vi "Update State.vi"(8 "error in (no error)":errorcluster, 10 "samples generated":i32, 11 "signal configuration":refnum<class "SV Discrete Sweep.lvclass">) -> (0 "error out":errorcluster, 1 "segment done":bool, 2 "generation done":bool, 3 "signal configuration":refnum<class "SV Discrete Sweep.lvclass">, 4 "measurement done":bool)   [LabVIEW 2017, in "SV Discrete Sweep.lvclass"]
uses:
  <vilib>/addons/_NISVFA/_Generation/Signal Generation/SV Discrete Sweep/SV Discrete Sweep.lvclass
  C:/Program Files (x86)/National Instruments/LabVIEW 2017/vi.lib/addons/_NISVFA/_Generation/Signal Generation/SV Signal/SV Signal.lvclass
  C:/Program Files (x86)/National Instruments/LabVIEW 2017/vi.lib/addons/_NISVFA/_Generation/Signal Generation/SV Function/SV Function.lvclass
  <vilib>/addons/_NISVFA/_Generation/Signal Generation/SV Signal/sv_Signal State Attribute.ctl
  <vilib>/addons/_NISVFA/_Generation/Signal Generation/SV Signal/sv_Generation State.ctl
  <vilib>/addons/_NISVFA/_Generation/Signal Generation/SV Discrete Sweep/SV Discrete Sweep.lvclass/SV Discrete Sweep.ctl
  <vilib>/addons/_NISVFA/_Generation/subVIs/sv_Optimum Location.ctl
  <vilib>/addons/_NISVFA/_Generation/Signal Generation/SV Signal/SV Signal.lvclass
  <vilib>/addons/_NISVFA/_Generation/Signal Generation/SV Signal/Read Transition Profile.vi
  <vilib>/addons/_NISVFA/_Generation/Signal Generation/SV Function/SV Function.lvclass
  <vilib>/addons/_NISVFA/_Generation/SoundVib_Generation.lvlib
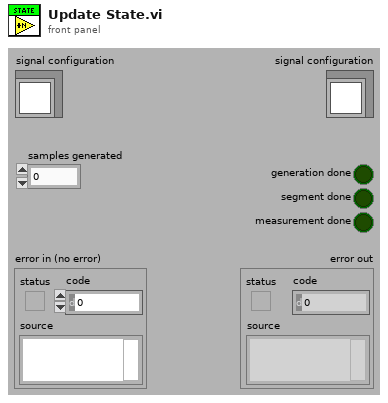
[diagram p1: front panel]
types:
  T1 = typedef "SV Signal.lvclass/sv_Signal State Attribute.ctl" = string
  T2 = typedef "SV Signal.lvclass/sv_Generation State.ctl" = enum16{"Idle", "Ramp Up", "Pre-Measurement Settling", "Measurement", "Post-Measurement Settling", "Discrete Sweep Transition", "Ramp Down", "Update"}
  T3 = typedef "SoundVib_Generation.lvlib/sv_Optimum Location.ctl" = enum16{"Zero Crossing, First Available", "Zero Crossing, Positive Slope", "Zero Crossing, Negative Slope", "Peak or Valley", "Peak", "Valley"}
  T4 = typedef "SV Signal.lvclass/sv_System Timing Model.ctl" = i64
  T5 = cluster{"system timing model":T4, "state":cluster{"RESET":bool, "generator timestamp":timestamp, "elapsed seconds":dbl, "elapsed samples":u64, "generation state":T2, "time offset at state":dbl, "samples generated at state":u64, "signal state":variant}, "duration of state":dbl, "samples remaining at state":i32}
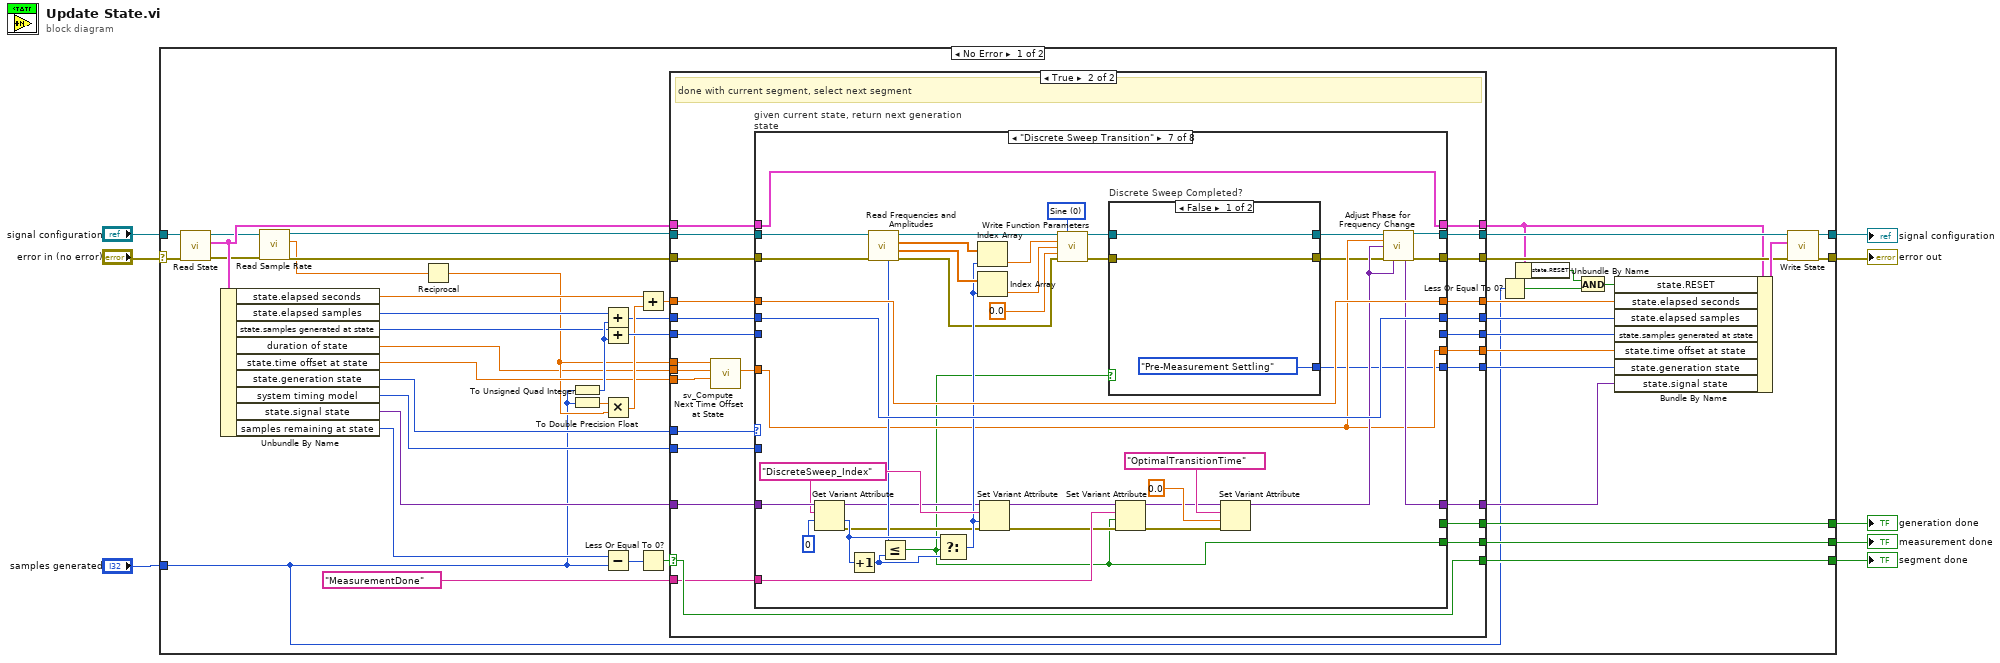
[diagram p0: block diagram]
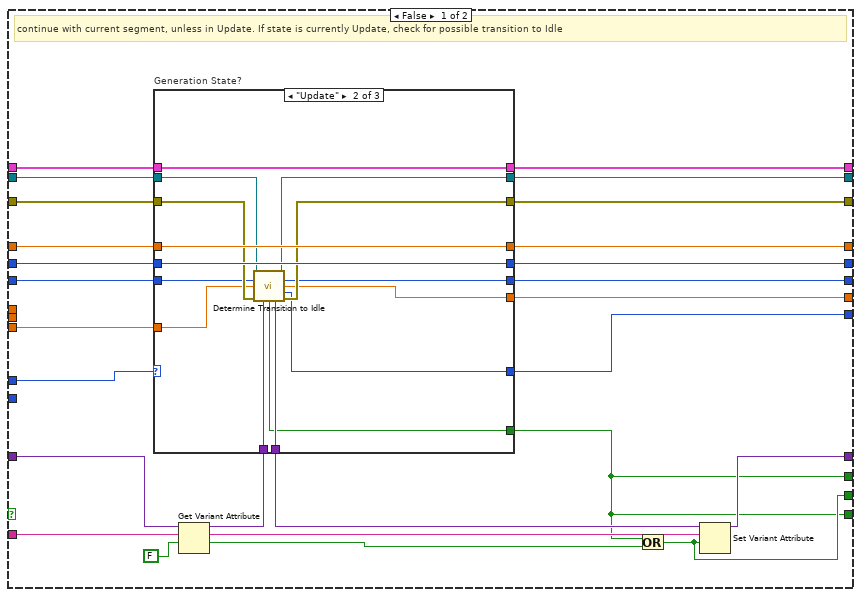
[diagram p2: hidden frame]
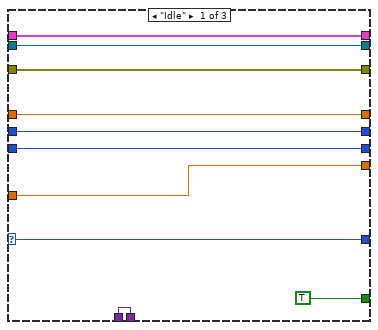
[diagram p3: hidden frame]
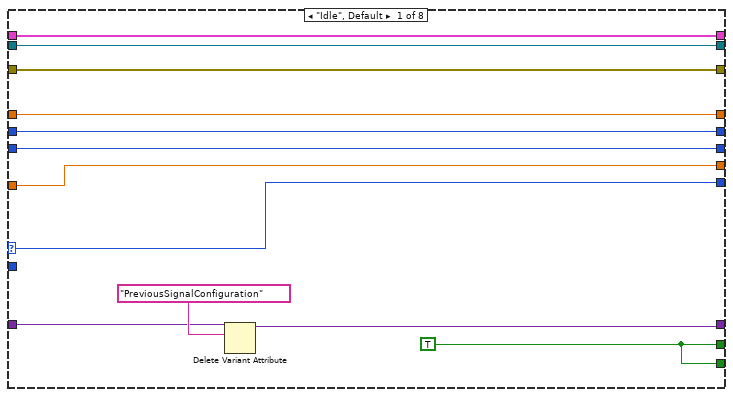
[diagram p5: hidden frame]
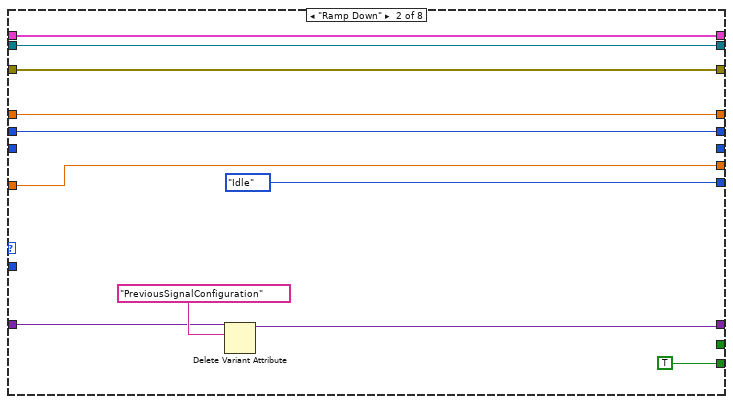
[diagram p6: hidden frame]
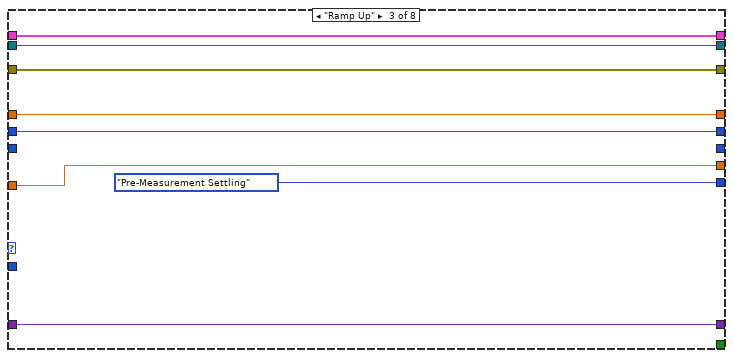
[diagram p7: hidden frame]
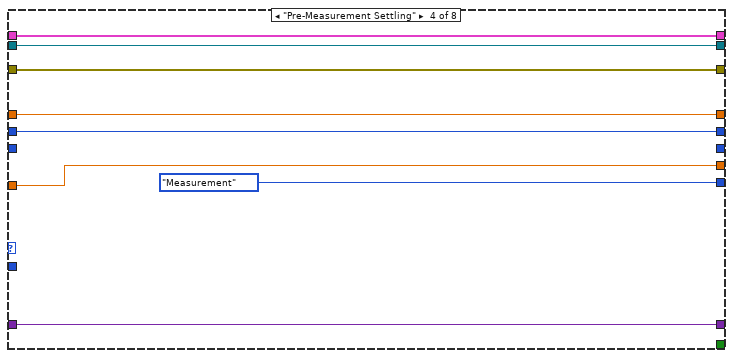
[diagram p8: hidden frame]
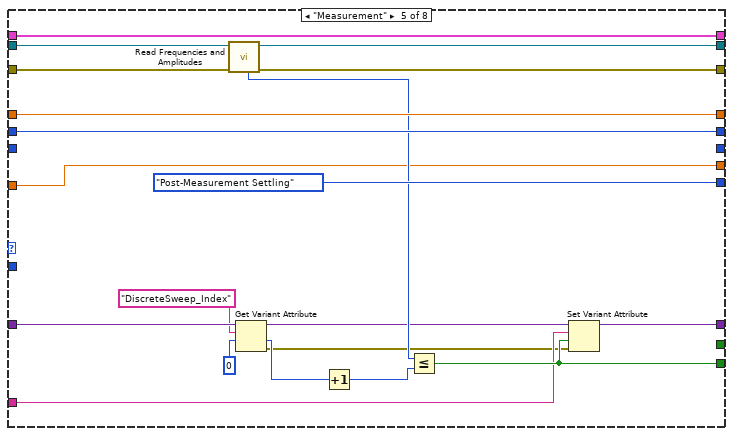
[diagram p9: hidden frame]
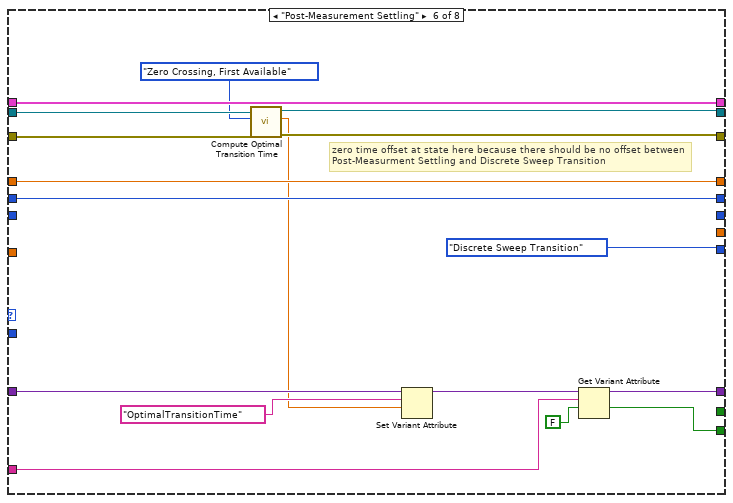
[diagram p10: hidden frame]
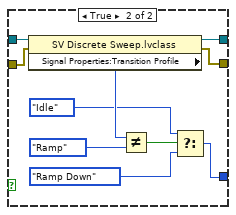
[diagram p11: hidden frame]
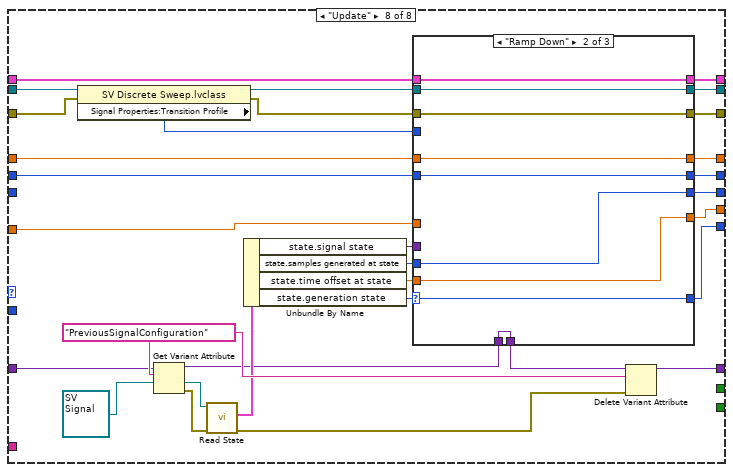
[diagram p12: hidden frame]
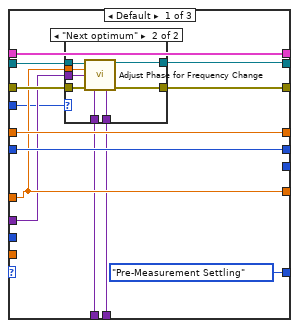
[diagram p13: hidden frame]
diagram:
  n1 = case shown="No Error" "error in (no error)" {
    selector: "error in (no error)" -> [w42 w341]
    tunnel: [w41 w341] -> w4
    tunnel: [w43 w342] -> w8
    tunnel: "signal configuration" -> [w45 w342]
    tunnel: "samples generated" -> [w9 _]
    tunnel: [w25 _] -> w3
    tunnel: [w46 _] -> w1
    tunnel: [w24 _] -> w2
    frame No Error {
      n2 = call <vilib>:"Read State.vi"("error in (no error)"=w42, "signal configuration"=w45) -> ("error out"=w19:errorcluster, "generator state"=w33:T5, "signal configuration"=w22:refnum<class "SV Discrete Sweep.lvclass">)  [unwired: 7 in]
      n3 = Unbundle By Name(w33) -> ("state.elapsed seconds"=w49:dbl, "state.elapsed samples"=w54:u64, "state.samples generated at state"=w39:u64, "duration of state"=w15:dbl, "state.time offset at state"=w17:dbl, "state.generation state"=w48:T2, "system timing model"=w47:T4, "state.signal state"=w36:variant, "samples remaining at state"=w26:i32)
      n4 = call <vilib>:"Read Sample Rate.vi"("error in (no error)"=w19, "signal configuration"=w22) -> ("error out"=w20:errorcluster, "sample rate [Hz]"=w18:dbl, "signal configuration"=w21:refnum<class "SV Discrete Sweep.lvclass">)  [unwired: 7 in]
      n5 = Reciprocal(x=w18) -> (1/x=w16:dbl)
      n6 = To Unsigned Quad Integer(1:w9) -> (0:w40:u64)
      n7 = To Double Precision Float(number=w9) -> (double precision float=w53:dbl)
      n8 = Add(x=w54, y=w40) -> (x+y=w31:u64)
      n9 = Add(x=w39, y=w40) -> (x+y=w38:u64)
      n10 = Multiply(x=w53, y=w16) -> (x*y=w37:dbl)
      n11 = Subtract(x=w26, y=w9) -> (x-y=w51:i32)
      n12 = Add(x=w49, y=w37) -> (x+y=w29:dbl)
      n13 = Less Or Equal To 0?(x=w51) -> (x <= 0?=w52:bool)
      n14 = case "done with segment?" shown="True" w52 {
        selector: w52 -> [_ w135]
        tunnel: [w56 w139] -> w35
        tunnel: w47 -> [_ w138]
        tunnel: w48 -> [w55 w137]
        tunnel: [w57 w136] -> w25
        tunnel: [w62 w120] -> w13
        tunnel: [w63 w119] -> w50
        tunnel: [w57 w135] -> w46
        tunnel: w38 -> [w65 w114]
        tunnel: w17 -> [w64 w115]
        tunnel: w36 -> [w79 w134]
        tunnel: [w78 w133] -> w34
        tunnel: w21 -> [w72 w132]
        tunnel: w33 -> [w73 w122]
        tunnel: w20 -> [w71 w130]
        tunnel: [w61 w126] -> w32
        tunnel: w31 -> [w66 w125]
        tunnel: [w60 w128] -> w30
        tunnel: w29 -> [w67 w127]
        tunnel: [w69 w131] -> w28
        tunnel: [w68 w121] -> w14
        tunnel: [w70 w129] -> w27
        tunnel: [w74 w124] -> w24
        tunnel: T1 "MeasurementDone" ("name") -> [w77 w123]
        tunnel: w16 -> [_ w117]
        tunnel: w15 -> [_ w116]
        frame False {
          # "continue with current segment, unless in Update. If state is currently Update, check for possible transition to Idle"
          n15 = Get Variant Attribute(Variant=w79, name=w77, default value (empty Variant)=FALSE) -> (duplicate Variant=w59:variant, value=w75:bool)  [unwired: 1 in, 2 out]
          n16 = case "Generation State?" shown="\"Update\"" w55 {
            selector: w55 -> [w80 _ w105]
            tunnel: [w89 w95 w113] -> w62
            tunnel: w65 -> [w89 w97 w113]
            tunnel: [w88 w94 w112] -> w63
            tunnel: w64 -> [w88 w96 w112]
            tunnel: [TRUE w90 _] -> w57
            tunnel: [w86 w100 w111] -> w69
            tunnel: w72 -> [w86 w101 w111]
            tunnel: [w85 w104 w110] -> w68
            tunnel: w73 -> [w85 w104 w110]
            tunnel: [w84 w98 w109] -> w70
            tunnel: w71 -> [w84 w99 w109]
            tunnel: [w83 w103 w108] -> w60
            tunnel: w67 -> [w83 w103 w108]
            tunnel: [w82 w102 w107] -> w61
            tunnel: w66 -> [w82 w102 w107]
            tunnel: w59 -> [w81 w93 w106]
            tunnel: [w81 w92 w106] -> w58
            tunnel: [w80 w91 w105] -> w56
            frame "Idle" {
            }
            frame "Update" {
              n17 = call <vilib>:"Determine Transition to Idle.vi"("SV Signal in"=w101, "samples generated at state in"=w97, "time offset at state in"=w96, "error in (no error)"=w99, "signal state in"=w93) -> ("SV Signal out"=w100:refnum<class "SV Discrete Sweep.lvclass">, "samples generated at state out"=w95:u64, "time offset at state out"=w94:dbl, "generation state out"=w91:T2, "transitioned to Idle?"=w90:bool, "signal state out"=w92:variant, "error out"=w98:errorcluster)  [unwired: 4 in]
            }
            frame Default {
            }
          }
          n18 = Or(x=w57, y=w75) -> (x .or. y?=w74:bool)
          n19 = Set Variant Attribute(Variant=w58, name=w77, value=w74) -> (Variant out=w78:variant)  [unwired: 1 in, 2 out]
        }
        frame True {
          # "done with current segment, select next segment"
          n20 = call <vilib>:"sv_Compute Next Time Offset at State.vi"("time offset at previous state"=w115, "duration of previous state"=w116, "dt"=w117) -> ("time offset at next state"=w118:dbl)  [unwired: 8 in]
          n21 = case "given current state, return next generation state" shown="\"Discrete Sweep Transition\"" w137 {
            selector: w137 -> [w141 _ _ _ _ _ _ _]
            tunnel: w138 -> [_ _ _ _ _ _ _ _]
            tunnel: [w141 sv_Generation_State."Idle" ("generation state") sv_Generation_State."Pre-Measurement Settling" ("generation state") sv_Generation_State."Measurement" ("generation state") sv_Generation_State."Post-Measurement Settling" ("generation state") sv_Generation_State."Discrete Sweep Transition" ("generation state") w216 w291] -> w139
            tunnel: [w147 _ _ _ _ _ _ _] -> w136
            tunnel: w134 -> [w145 w155 w169 w177 w197 w202 w255 w296]
            tunnel: [w144 w154 w169 w177 w194 w212 w225 w299] -> w133
            tunnel: w132 -> [w151 w161 w168 w176 w187 w208 w223 w273]
            tunnel: [w151 w161 w168 w176 w186 w207 w228 w284] -> w131
            tunnel: w130 -> [w150 w160 w167 w175 w185 w206 w222 w272]
            tunnel: [w150 w160 w167 w175 w184 w205 w227 w283] -> w129
            tunnel: [w149 w159 w166 w174 w196 w214 w253 w281] -> w128
            tunnel: w127 -> [w149 w159 w166 w174 w196 w214 w253 w282]
            tunnel: [w148 w158 w165 w173 w195 w213 w252 w280] -> w126
            tunnel: w125 -> [w148 w158 w165 w173 w195 w213 w252 w279]
            tunnel: [w147 TRUE _ _ w193 w209 w221 _] -> w124
            tunnel: w123 -> [_ _ _ _ w192 w211 w251 _]
            tunnel: w122 -> [w143 w153 w164 w172 w180 w204 w233 w285]
            tunnel: [w143 w153 w164 w172 w180 w204 w233 w286] -> w121
            tunnel: [w140 _ _ _ _ _ _ w292] -> w120
            tunnel: [w142 w152 w163 w171 w179 _ w224 w288] -> w119
            tunnel: w118 -> [w142 w152 w163 w171 w179 _ w224 w287]
            tunnel: w114 -> [w140 _ _ _ _ _ _ _]
            frame "Idle", Default {
              w147 = TRUE
              n22 = Delete Variant Attribute(6:T1 "PreviousSignalConfiguration" ("name (all attributes)"), 7:w145) -> (3:w144:variant)  [unwired: 1 in, 2 out]
            }
            frame "Ramp Down" {
              n23 = Delete Variant Attribute(6:T1 "PreviousSignalConfiguration" ("name (all attributes)"), 7:w155) -> (3:w154:variant)  [unwired: 1 in, 2 out]
            }
            frame "Ramp Up" {
            }
            frame "Pre-Measurement Settling" {
            }
            frame "Measurement" {
              n24 = call <vilib>:"Read Frequencies and Amplitudes.vi"("error in (no error)"=w185, "SV Discrete Sweep in"=w187) -> ("error out"=w184:errorcluster, "SV Discrete Sweep out"=w186:refnum<class "SV Discrete Sweep.lvclass">, "number of steps"=w183:i32)  [unwired: 5 in, 2 out]
              n25 = Get Variant Attribute(Variant=w197, name="DiscreteSweep_Index", default value (empty Variant)=0 ("samples generated")) -> (duplicate Variant=w182:variant, value=w190:i32, error out=w181:errorcluster)  [unwired: 1 in, 1 out]
              n26 = Increment(x=w190) -> (x+1=w189:i32)
              n27 = Less Or Equal?(x=w183, y=w189) -> (x <= y?=w193:bool)
              n28 = Set Variant Attribute(Variant=w182, name=w192, value=w193, error in=w181) -> (Variant out=w194:variant)  [unwired: 2 out]
            }
            frame "Post-Measurement Settling" {
              # "zero time offset at state here because there should be no offset between Post-Measurment Settling and Discrete Sweep Transition"
              n29 = call-dynamic "Compute Optimal Transition Time.vi"("error in (no error)"=w206, "optimum"=sv_Optimum_Location."Zero Crossing, First Available", "SV Function in"=w208) -> ("error out"=w205:errorcluster, "optimal transition time"=w200:dbl, "SV Function out"=w207:refnum<class "SV Discrete Sweep.lvclass">)  [unwired: 6 in]
              n30 = Set Variant Attribute(Variant=w202, name=T1 "OptimalTransitionTime" ("attribute"), value=w200) -> (Variant out=w201:variant)  [unwired: 1 in, 2 out]
              n31 = Get Variant Attribute(Variant=w201, name=w211, default value (empty Variant)=FALSE ("found")) -> (duplicate Variant=w212:variant, value=w209:bool)  [unwired: 1 in, 2 out]
            }
            frame "Discrete Sweep Transition" {
              w246 = u16 0 items=["Sine", "Triangle", "Square", "Sawtooth"] ("function type")
              w247 = T1 "DiscreteSweep_Index" ("name")
              n32 = Get Variant Attribute(Variant=w255, name=w247, default value (empty Variant)=0 ("samples generated")) -> (duplicate Variant=w235:variant, value=w249:i32, error out=w234:errorcluster)  [unwired: 1 in, 1 out]
              n33 = Increment(x=w249) -> (x+1=w248:i32)
              n34 = call <vilib>:"Read Frequencies and Amplitudes.vi"("error in (no error)"=w222, "SV Discrete Sweep in"=w223) -> ("error out"=w238:errorcluster, "amplitudes"=w242:dbl[], "frequencies_Hz"=w243:dbl[], "SV Discrete Sweep out"=w245:refnum<class "SV Discrete Sweep.lvclass">, "number of steps"=w236:i32)  [unwired: 5 in]
              n35 = Less Or Equal?(x=w236, y=w248) -> (x <= y?=w221:bool)
              n36 = Select(t=w249, s=w221, f=w248) -> (s? t:f=w241:i32)
              n37 = Index Array(array=w243, index=w241) -> (element=w240:dbl)
              n38 = Index Array(array=w242, index=w241) -> (element=w239:dbl)
              n39 = Set Variant Attribute(Variant=w235, name=w247, value=w241, error in=w234) -> (Variant out=w254:variant, error out=w237:errorcluster)  [unwired: 1 out]
              n40 = call <vilib>:"Write Function Parameters.vi"("signal configuration"=w245, "function type"=w246, "frequency (Hz)"=w240, "amplitude"=w239, "phase (deg)"=0.0, "error in (no error)"=w238) -> ("signal configuration"=w220:refnum<class "SV Discrete Sweep.lvclass">, "error out"=w217:errorcluster)  [unwired: 8 in]
              n41 = case "Discrete Sweep Completed?" shown="False" w221 {
                tunnel: w220 -> [w258 w268]
                tunnel: [w258 w267] -> w219
                tunnel: [w257 w265] -> w218
                tunnel: w217 -> [w257 w266]
                tunnel: [sv_Generation_State."Pre-Measurement Settling" ("generation state") w260] -> w216
                frame False {
                }
                frame True {
                  n42 = property class="SV Discrete Sweep.lvclass"(reference=w268, error in=w266) -> (reference out=w267:refnum<class "SV Discrete Sweep.lvclass">, error out=w265:errorcluster, "Signal Properties:Transition Profile"=w264:enum16{"Immediate", "Next optimum", "Ramp"})
                  n43 = Not Equal?(x=w264, y=enum16{"Immediate", "Next optimum", "Ramp"}."Ramp") -> (x != y?=w259:bool)
                  n44 = Select(t=sv_Generation_State."Idle" ("generation state"), s=w259, f=sv_Generation_State."Ramp Down" ("generation state")) -> (s? t:f=w260:T2)
                }
              }
              n45 = Set Variant Attribute(Variant=w254, name=w251, value=w221, error in=w237) -> (Variant out=w230:variant, error out=w229:errorcluster)  [unwired: 1 out]
              n46 = Set Variant Attribute(Variant=w230, name=T1 "OptimalTransitionTime" ("attribute"), value=0.0 ("phase (deg)"), error in=w229) -> (Variant out=w226:variant)  [unwired: 2 out]
              n47 = call <vilib>:"Adjust Phase for Frequency Change.vi"("SV Signal in"=w219, "time offset at state"=w224, "previous signal state"=w226, "error in (no error)"=w218, "signal state in"=w226) -> ("SV Signal out"=w228:refnum<class "SV Discrete Sweep.lvclass">, "signal state out"=w225:variant, "error out"=w227:errorcluster)  [unwired: 8 in]
            }
            frame "Update" {
              w297 = T1 "PreviousSignalConfiguration" ("name (all attributes)")
              n48 = property class="SV Discrete Sweep.lvclass"(reference=w273, error in=w272) -> (reference out=w270:refnum<class "SV Discrete Sweep.lvclass">, error out=w271:errorcluster, "Signal Properties:Transition Profile"=w269:enum16{"Immediate", "Next optimum", "Ramp"})
              n49 = Get Variant Attribute(Variant=w296, name=w297, default value (empty Variant)=refnum<class "SV Signal.lvclass"> refnum ("signal configuration")) -> (duplicate Variant=w275:variant, value=w295:refnum<class "SV Signal.lvclass">, error out=w278:errorcluster)  [unwired: 1 in, 1 out]
              n50 = call <vilib>:"Read State.vi"("error in (no error)"=w278, "signal configuration"=w295) -> ("error out"=w277:errorcluster, "generator state"=w294:T5)  [unwired: 7 in, 1 out]
              n51 = Unbundle By Name(w294) -> ("state.signal state"=w276:variant, "state.samples generated at state"=w289:u64, "state.time offset at state"=w290:dbl, "state.generation state"=w293:T2)
              n52 = case shown="\"Ramp Down\"" w293 {
                selector: w293 -> [_ w332 w340]
                tunnel: [sv_Generation_State."Pre-Measurement Settling" ("generation state") w332 w340] -> w291
                tunnel: [_ w331 _] -> w292
                tunnel: w290 -> [_ w330 _]
                tunnel: w289 -> [_ w331 _]
                tunnel: [w304 w330 w339] -> w288
                tunnel: w287 -> [w304 _ w339]
                tunnel: [w309 w329 w334] -> w286
                tunnel: w285 -> [w309 w329 w334]
                tunnel: [w307 w328 w335] -> w284
                tunnel: w270 -> [w308 w328 w335]
                tunnel: [w305 w327 w336] -> w283
                tunnel: w271 -> [w306 w327 w336]
                tunnel: [w310 w326 w337] -> w281
                tunnel: w282 -> [w310 w326 w337]
                tunnel: [w311 w325 w338] -> w280
                tunnel: w279 -> [w311 w325 w338]
                tunnel: w276 -> [w303 _ _]
                tunnel: w275 -> [w302 w324 w333]
                tunnel: [w301 w324 w333] -> w274
                tunnel: w269 -> [w300 _ _]
                frame Default {
                  n53 = case shown="\"Next optimum\"" w300 {
                    tunnel: w308 -> [w315 w323]
                    tunnel: [w315 w322] -> w307
                    tunnel: w306 -> [w314 w321]
                    tunnel: [w314 w320] -> w305
                    tunnel: w304 -> [_ w319]
                    tunnel: w303 -> [_ w318]
                    tunnel: w302 -> [w313 w317]
                    tunnel: [w313 w316] -> w301
                    frame "Immediate", Default {
                    }
                    frame "Next optimum" {
                      n54 = call <vilib>:"Adjust Phase for Frequency Change.vi"("SV Signal in"=w323, "time offset at state"=w319, "previous signal state"=w318, "error in (no error)"=w321, "signal state in"=w317) -> ("SV Signal out"=w322:refnum<class "SV Discrete Sweep.lvclass">, "signal state out"=w316:variant, "error out"=w320:errorcluster)  [unwired: 8 in]
                    }
                  }
                }
                frame "Ramp Down" {
                }
                frame "Idle" {
                }
              }
              n55 = Delete Variant Attribute(4:w277, 6:w297, 7:w274) -> (3:w299:variant)  [unwired: 2 out]
            }
          }
        }
      }
      n56 = Less Or Equal To 0?(x=w9) -> (x <= 0?=w11:bool)
      n57 = Unbundle By Name(w14) -> ("state.RESET"=w12:bool)
      n58 = And(x=w12, y=w11) -> (x .and. y?=w10:bool)
      n59 = Bundle By Name(cluster=w14, "state.RESET"=w10, "state.elapsed seconds"=w30, "state.elapsed samples"=w32, "state.samples generated at state"=w13, "state.time offset at state"=w50, "state.generation state"=w35, "state.signal state"=w34) -> (w44:T5)
      n60 = call <vilib>:"Write State.vi"("error in (no error)"=w27, "generator state"=w44, "signal configuration"=w28) -> ("error out"=w41:errorcluster, "signal configuration"=w43:refnum<class "SV Discrete Sweep.lvclass">)  [unwired: 7 in]
    }
    frame Error {
    }
  }
  "error out" <- w4
  "signal configuration" <- w8
  "generation done" <- w3
  "segment done" <- w1
  "measurement done" <- w2
